vi "Neocera21 Get T and H.vi"(8 "error in (no error)":errorcluster, 10 "Private data":T1={"Channels to measure"=[1.0], "Record heater"=FALSE, "Set point"=0.0, "Set Heater Range"=enum."Off", "Control"=FALSE, "Approach"=enum."Instant", "Ramp rate, K/min"=1.0, "Control Channel"=1, "P"=0.0, "I"=0.0, "D"=0.0, "Suspend heater"=FALSE}, 11 "VISA Resource Name":refnum<visa-resource-name>) -> (0 "error out":errorcluster, 1 "data string":string, 2 "Data out":dbl[](array[numeric]), 3 "VISA Resource Name Out":refnum<visa-resource-name>, 4 "Heat %":dbl format="%.2f")   [LabVIEW 2015]
uses:
  Neocera Front Panel Data.ctl
  Neocera Heater Ranges.ctl
  Neocera Set Point Aproach.ctl
panel:
  # "Temperature Monitor"
  # "Temperature Control"
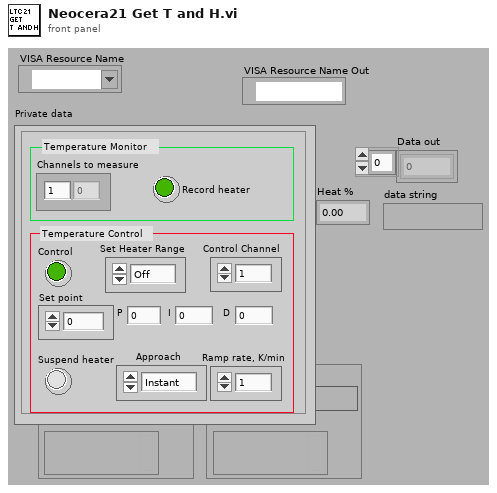
[diagram p1: front panel]
types:
  T1 = typedef "Neocera Front Panel Data.ctl" = cluster{"Channels to measure":dbl[], "Record heater":bool, "Set point":dbl, "Set Heater Range":T2, "Control":bool, "Approach":T3, "Ramp rate, K/min":dbl, "Control Channel":i16, "P":dbl, "I":dbl, "D":dbl, "Suspend heater":bool}
  T2 = typedef "Neocera Heater Ranges.ctl" = enum16{"Off", "0.05W", "0.5W", "5W", "50W"}
  T3 = typedef "Neocera Set Point Aproach.ctl" = enum16{"Instant", "Ramp"}
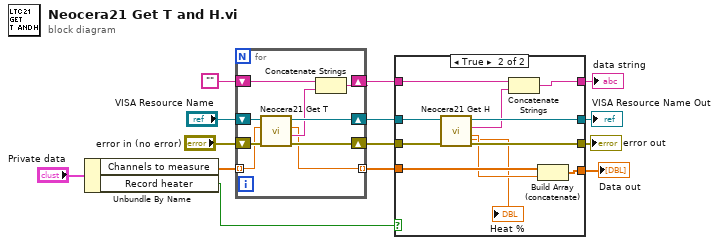
[diagram p0: block diagram]
diagram:
  n1 = Unbundle By Name("Private data") -> ("Channels to measure"=w11:dbl[], "Record heater"=w9:bool)
  n2 = for {
    shift-right: [w21] -> w6
    shift-left: "VISA Resource Name" -> [w22]
    shift-right: [w23] -> w8
    shift-left: "error in (no error)" -> [w16]
    tunnel: w11 -> [w15] mode=indexing
    tunnel: [w17] -> w2 mode=indexing
    shift-right: [w19] -> w4
    shift-left: "" -> [w20]
    n3 = call "Neocera21 Get T.vi"("error in (no error)"=w16, "Sensor"=w15, "VISA Resource Name"=w22) -> ("error out"=w23:errorcluster, "data string"=w18:string, "Temperature"=w17:dbl, "VISA Resource Name Out"=w21:refnum<visa-resource-name>)  [unwired: 5 in]
    n4 = Concatenate Strings(w20, w18) -> (w19:string)
  }
  n5 = case shown="True" w9 {
    tunnel: w8 -> [w27 w30]
    tunnel: [w27 w38] -> w7
    tunnel: w6 -> [w26 w31]
    tunnel: [w26 w37] -> w5
    tunnel: w4 -> [w25 w36]
    tunnel: [w25 w34] -> w3
    tunnel: w2 -> [w24 w33]
    tunnel: [w24 w32] -> w1
    frame False {
    }
    frame True {
      n6 = call "Neocera21 Get H.vi"("error in (no error)"=w30, "VISA Resource Name"=w31) -> ("error out"=w38:errorcluster, "Heater power"=w29:dbl, "data string"=w35:string, "VISA Resource Name Out"=w37:refnum<visa-resource-name>, "Heat %"=→"Heat %":dbl)  [unwired: 4 in, 1 out]
      n7 = Concatenate Strings(w36, w35) -> (w34:string)
      n8 = Build Array (concatenate)(w33, w29) -> (w32:dbl[])
    }
  }
  "error out" <- w7
  "data string" <- w3
  "Data out" <- w1
  "VISA Resource Name Out" <- w5
